vi "Create DUT Setup Step Reference.vi"(8 "error in (no error)":errorcluster, 11 "QPA Measurement in":refnum<class "QPA Measurement.lvclass">) -> (0 "error out":errorcluster, 3 "QPA Measurement out":refnum<class "QPA Measurement.lvclass">)   [LabVIEW 2016, in "QPA Measurement.lvlib" / "QPA Measurement.lvclass"]
uses:
  QPA Measurement.lvclass
  C:/Sequence Automation/Plugins/Measurement Interface.lvlibp/Measurement Interface.lvclass
  QPA Measurement.lvclass/QPA Measurement.ctl
  Plugins/Measurement Interface.lvlibp/Private Methods/Engine Reference/Read Engine Reference.vi
  Plugins/Measurement Interface.lvlibp/Private Methods/Active Sequence File/Read Active Sequence File.vi
  Plugins/TestStand API Tools (TSAT).lvlibp/Step Actions/TSAT Step Actions.lvlib
  Plugins/TestStand API Tools (TSAT).lvlibp/Sequence File Actions/TSAT Sequence File Actions.lvlib
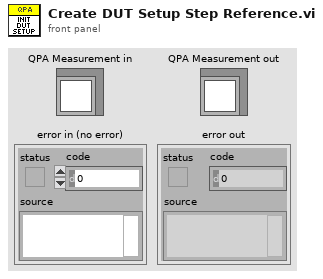
[diagram p1: front panel]
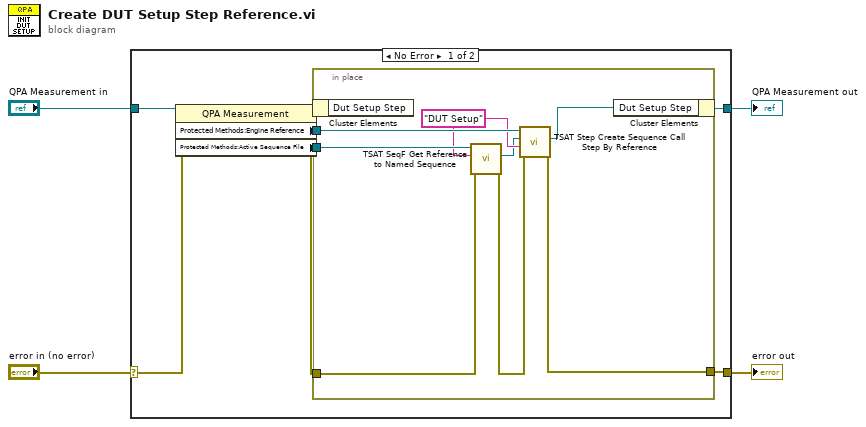
[diagram p0: block diagram]
diagram:
  n1 = case shown="No Error" "error in (no error)" {
    selector: "error in (no error)" -> [w11 w22]
    tunnel: [w6 w22] -> w3
    tunnel: [w12 w21] -> w1
    tunnel: "QPA Measurement in" -> [w9 w21]
    frame No Error {
      n2 = property class="QPA Measurement"(reference=w9, error in=w11) -> (reference out=w8:refnum<class "QPA Measurement.lvclass">, error out=w10:errorcluster, "Protected Methods:Engine Reference"=w7:refnum<k7>, "Protected Methods:Active Sequence File"=w5:refnum<k7>)
      n3 = in-place {
        in-place-border: w10 -> [w14]
        in-place-border: w7 -> [w20]
        in-place-border: [w19] -> w6
        in-place-border: w5 -> [w17]
        w16 = "DUT Setup" ("Step Name")
        n4 = in-place-cluster #1(w8) -> ()  [unwired: 1 out]
        n5 = call "TSAT SeqF Get Reference to Named Sequence.vi"("Error In"=w14, "Seqeunce to Retrieve"=w16, "Sequence File In"=w17) -> ("Error Out"=w13:errorcluster, "Named Sequence"=w15:refnum<k7>)  [unwired: 6 in, 1 out]
        n6 = call "TSAT Step Create Sequence Call Step By Reference.vi"("Error In"=w13, "Step Name"=w16, "Sequence to Call"=w15, "Engine In"=w20) -> ("Error Out"=w19:errorcluster, "Step Reference"=w18:refnum<k7>)  [unwired: 5 in, 1 out]
        n7 = in-place-cluster #1("Dut Setup Step"=w18) -> (w12:refnum<class "QPA Measurement.lvclass">)
      }
    }
    frame Error {
    }
  }
  "error out" <- w3
  "QPA Measurement out" <- w1
